vi "BRig_RT__Case_Exp__comm_tcp__data_analog__PortA.vi"(5 "input_AI0":u16, 7 "input_AI1":u16, 8 "input_strAccum":string, 9 "input_error":errorcluster, 10 "input_hTCP":refnum<k5>, 11 "input_I_connected_TCP":bool) -> (0 "output_strAccum":string, 1 "output_error":errorcluster, 2 "output_hTCP":refnum<k5>, 3 "output_I_connect_TCP":bool)   [LabVIEW 2014]
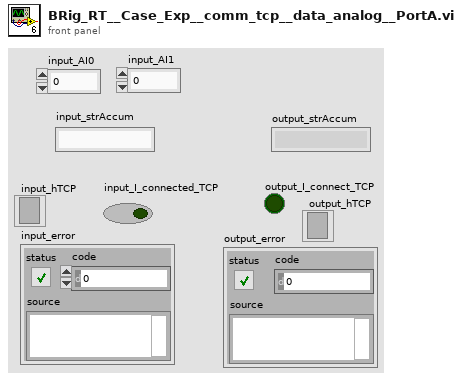
[diagram p1: front panel]
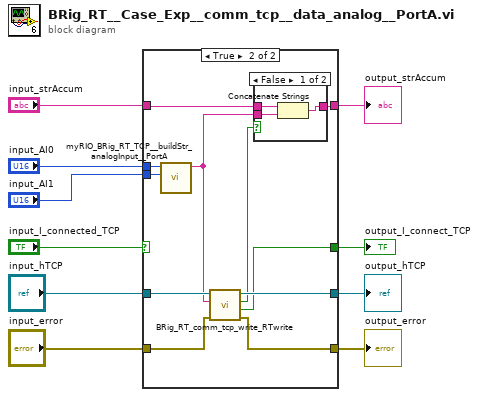
[diagram p0: block diagram]
diagram:
  n1 = case shown="True" "input_I_connected_TCP" {
    selector: "input_I_connected_TCP" -> [w12 _]
    tunnel: "input_hTCP" -> [w14 w23]
    tunnel: "input_error" -> [w13 w22]
    tunnel: "input_AI0" -> [_ w25]
    tunnel: "input_AI1" -> [_ w24]
    tunnel: [w14 w21] -> w2
    tunnel: [w13 w20] -> w1
    tunnel: [w12 w19] -> w3
    tunnel: "input_strAccum" -> [w11 w18]
    tunnel: [w11 w16] -> w4
    frame False {
    }
    frame True {
      n2 = call "myRIO_BRig_RT_TCP__buildStr_analogInput__PortA.vi"("input_AI1"=w24, "input_AI0"=w25) -> ("output_str_analogInput"=w17:string)  [unwired: 9 in]
      n3 = call "BRig_RT_comm_tcp_write_RTwrite.vi"("input_error"=w22, "input_packet"=w17, "input_hTCP"=w23) -> ("output_error"=w20:errorcluster, "output_I_NotDisconnected"=w19:bool, "output_I_write"=w15:bool, "output_hTCP"=w21:refnum<k5>)  [unwired: 5 in]
      n4 = case shown="False" w15 {
        tunnel: w18 -> [w28 w29]
        tunnel: w17 -> [w27 _]
        tunnel: [w26 w29] -> w16
        frame False {
          n5 = Concatenate Strings(w28, w27) -> (w26:string)
        }
        frame True {
        }
      }
    }
  }
  "output_strAccum" <- w4
  "output_I_connect_TCP" <- w3
  "output_hTCP" <- w2
  "output_error" <- w1
